vi "coordinate_locator.vi"(10 "Shape Cluster":T1, 11 "Dimensions":T2) -> (2 "y coord":i32, 3 "x coord":i32)   [LabVIEW 2015]
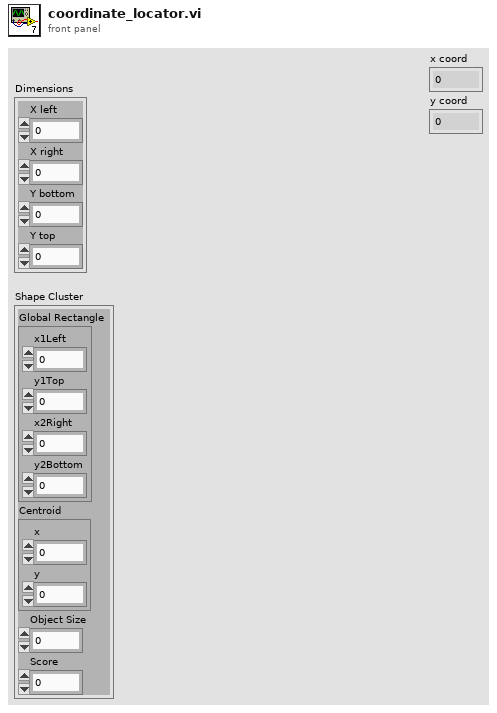
[diagram p1: front panel]
types:
  T1 = cluster{"Global Rectangle":cluster{"x1Left":i32, "y1Top":i32, "x2Right":i32, "y2Bottom":i32}, "Centroid":cluster{"x":sgl, "y":sgl}, "Object Size":u32, "Score":dbl}
  T2 = cluster{"X left":dbl, "X right":dbl, "Y bottom":dbl, "Y top":dbl}
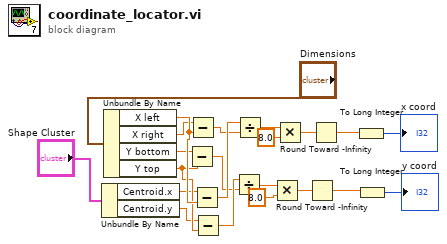
[diagram p0: block diagram]
diagram:
  n1 = Unbundle By Name("Shape Cluster") -> ("Centroid.x"=w17:sgl, "Centroid.y"=w18:sgl)
  n2 = Unbundle By Name("Dimensions") -> ("X left"=w20:dbl, "X right"=w9:dbl, "Y bottom"=w7:dbl, "Y top"=w19:dbl)
  n3 = Subtract(x=w7, y=w19) -> (x-y=w8:dbl)
  n4 = Subtract(x=w9, y=w20) -> (x-y=w10:dbl)
  n5 = Subtract(x=w17, y=w20) -> (x-y=w21:dbl)
  n6 = Subtract(x=w18, y=w19) -> (x-y=w22:dbl)
  n7 = Divide(x=w22, y=w8) -> (x/y=w11:dbl)
  n8 = Divide(x=w21, y=w10) -> (x/y=w14:dbl)
  n9 = Multiply(x=w11, y=8.0) -> (x*y=w13:dbl)
  n10 = Multiply(x=w14, y=8.0) -> (x*y=w16:dbl)
  n11 = Round Toward -Infinity(1:w13) -> (0:w3:dbl)
  n12 = Round Toward -Infinity(1:w16) -> (0:w4:dbl)
  n13 = To Long Integer(number=w4) -> (32bit integer=→"x coord":i32)
  n14 = To Long Integer(number=w3) -> (32bit integer=→"y coord":i32)
